vi "Write.vi"(8 "error in (no error)":errorcluster {"code" format="%.0x"}, 10 "Write Buffer":string, 11 "VISA resource name":refnum<visa-resource-name>) -> (0 "error out":errorcluster {"code" format="%.0x"}, 3 "VISA resource name out":refnum<visa-resource-name>)   [LabVIEW 2014, in "Fluke 190 Series II.lvlib"]
doc: "Replaces LabVIEW VISA Write. For each write command, a carriage return constant appened to the end, and an acknowledge value is returned, which indicates correct or incorrect operation."
uses:
  Fluke 190 Series II.lvlib
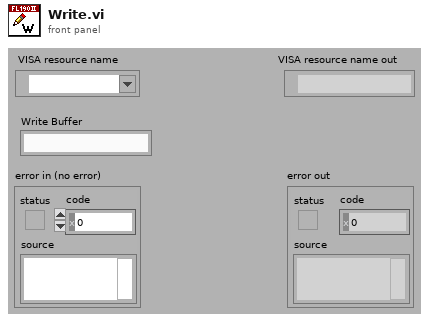
[diagram p1: front panel]
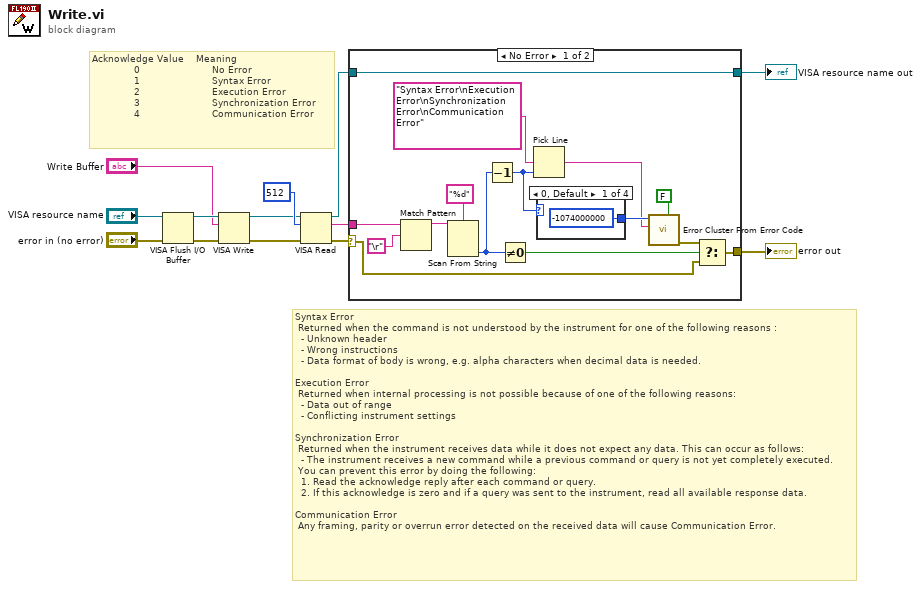
[diagram p0: block diagram]
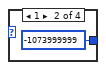
[diagram p2: hidden frame]
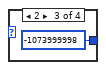
[diagram p3: hidden frame]
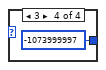
[diagram p4: hidden frame]
diagram:
  # "Acknowledge Value    Meaning\n              0                        No Error\n              1                        Syntax Error\n              2                        Execution Error\n              3                        Synchronization Error\n              4                        Communication Error"
  # "Syntax Error\n Returned when the command is not understood by the instrument for one of the following reasons :\n  - Unknown header\n  - Wrong instructions\n  - Data format of body is wrong, e.g. alpha characters when decimal data is needed.\n\nExecution Error\n Returned when internal processing is not possible because of one of the following reasons:\n  - Data out of range\n  - Conflicting instrument settings\n\nSynchronization Error\n Returned when the instrument receives data while it does not expect any data. This can occur as follows:\n  - The instrument receives a new command while a previous command or query is not yet completely executed.\n You can prevent this error by doing the following:\n  1. Read the acknowledge reply after each command or query.\n  2. If this acknowledge is zero and if a query was sent to the instrument, read all available response data.\n\nCommunication Error\n Any framing, parity or overrun error detected on the received data will cause Communication Error."
  n1 = VISA Flush I/O Buffer(VISA resource name="VISA resource name", error in (no error)="error in (no error)") -> (VISA resource name out=w11:refnum<visa-resource-name>, error out=w10:errorcluster)  [unwired: 1 out]
  n2 = VISA Write(VISA resource name=w11, write buffer="Write Buffer", error in (no error)=w10) -> (VISA resource name out=w3:refnum<visa-resource-name>, error out=w2:errorcluster)  [unwired: 1 out]
  n3 = VISA Read(VISA resource name=w3, byte count=u32 512, error in (no error)=w2) -> (VISA resource name out=w8:refnum<visa-resource-name>, read buffer=w7:string, error out=w6:errorcluster)  [unwired: 1 out]
  n4 = case shown="No Error" w6 {
    selector: w6 -> [w23 w34]
    tunnel: w7 -> [w28 _]
    tunnel: w8 -> [w14 w33]
    tunnel: [w22 w34] -> w5
    tunnel: [w14 w33] -> w4
    frame No Error {
      n5 = Match Pattern(string=w28, regular expression="\r") -> (before substring=w26:string)  [unwired: 4 out]
      n6 = Scan From String(format string="%d", input string=w26) -> (output 1=w19:i32)  [unwired: 2 in, 4 out]
      n7 = Decrement(x=w19) -> (x-1=w17:i32)
      n8 = Not Equal To 0?(x=w19) -> (x != 0?=w24:bool)
      n9 = Pick Line(multi-line string="Syntax Error\nExecution Error\nSynchronization Error\nCommunication Error", line index=w17) -> (output string=w15:string)  [unwired: 1 out]
      n10 = case shown="0, Default" w17 {
        tunnel: [-1074000000 -1073999999 -1073999998 -1073999997] -> w16
        frame 0, Default {
        }
        frame 1 {
        }
        frame 2 {
        }
        frame 3 {
        }
      }
      n11 = call <vilib>:"Error Cluster From Error Code.vi"("is warning? (False)"=FALSE, "error message (\"\")"=w15, "error code (0)"=w16) -> ("error out"=w20:errorcluster)  [unwired: 2 in, 4 out]
      n12 = Select(t=w20, s=w24, f=w23) -> (s? t:f=w22:errorcluster)
    }
    frame Error {
    }
  }
  "error out" <- w5
  "VISA resource name out" <- w4
